vi "创建数组.vi"() -> ()   [LabVIEW 2018]
panel:
  out "最小值":dbl
  out "最大值":dbl
  out "添加的数组":dbl[](array[numeric])
  out "元素 3":dbl
  out "元素 2":dbl
  out "元素":dbl
  out "数组":dbl[](array[numeric])
  out "大小":i32
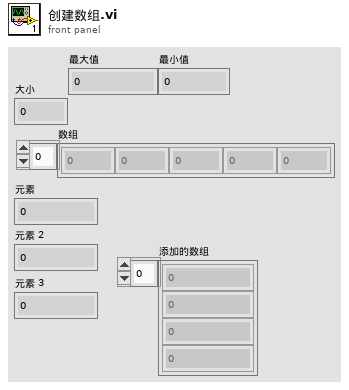
[diagram p1: front panel]
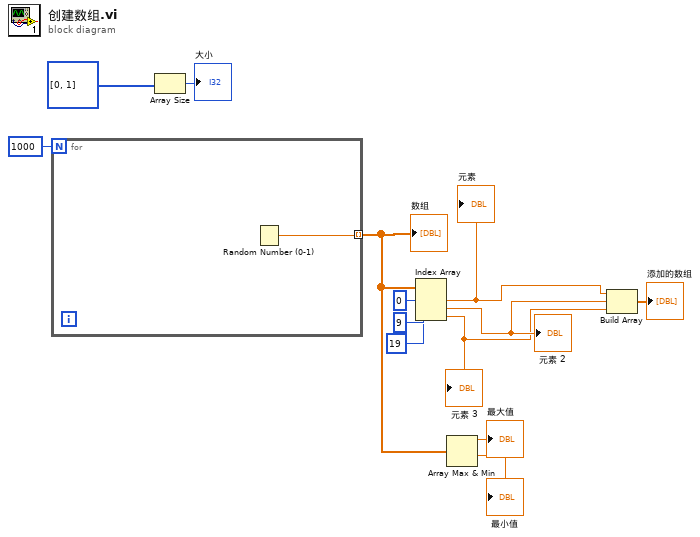
[diagram p0: block diagram]
diagram:
  n1 = for {
    N: 1000 -> [_]
    tunnel: [w14] -> w3 mode=indexing
    n2 = Random Number (0-1)() -> (number: 0 to 1=w14:dbl)
  }
  "数组" <- w3
  n3 = Array Size(array=i32[] [0, 1]) -> (size(s)=→"大小":i32)
  n4 = Index Array(array=w3, index #1=0 ("索引"), index #2=9 ("索引"), index #3=19 ("索引")) -> (element #1=w7:dbl, element #2=w6:dbl, element #3=w5:dbl)
  "元素" <- w7
  "元素 2" <- w6
  "元素 3" <- w5
  n5 = Array Max & Min(array=w3) -> (max value=→"最大值":dbl, min value=→"最小值":dbl)  [unwired: 2 out]
  n6 = Build Array(w7, w6, w5) -> (→"添加的数组":dbl[])
